vi "Set One Test.vi"() -> ()   [LabVIEW 2018]
doc: "Use this template to build a user interface event handler design pattern. Use this pattern for dialog boxes and other user interfaces. You also can create and execute user-defined events that the VI can handle the same way as user interface events."
uses:
  Private/Types/MALT CardTypes.ctl
panel:
  in  "State":bool
  in  "Port":i32=4
  in  "Address":i32=3
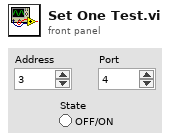
[diagram p1: front panel]
types:
  T1 = typedef "MALT CardTypes.ctl" = enum32{"-", "YAV90832", "YAV904X8", "MALT132", "YAV91616", "YAV90PIN", "YAV90096", "YAV90HVT", "YAV90CLR", "YAV90128", "YAV90PNE", "YAVCANCON", "YAV91775", "YAV90XXX", "YAV90MMU", "H730050", "H710060", "H710061", "YAV90304", "MMI", "YAV90060", "MALT160T", "YAV90059", "Not Defined"}
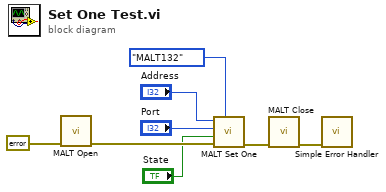
[diagram p0: block diagram]
diagram:
  n1 = call "MALT Open.vi"("error in"=errorcluster {"status"=FALSE, "code"=0, "source"=""}) -> ("error out"=w8:errorcluster)  [unwired: 10 in]
  n2 = call "MALT Set One.vi"("MALT FamilyCode"=MALT_CardTypes."MALT132" ("MALT CardType"), "error in"=w8, "State"="State", "Relay Num"="Port", "Address"="Address") -> ("error out"=w2:errorcluster)  [unwired: 5 in]
  n3 = call "MALT Close.vi"("error in"=w2) -> ("error out"=w6:errorcluster)  [unwired: 10 in]
  n4 = call <vilib>:"Simple Error Handler.vi"("error in (no error)"=w6) -> ()  [unwired: 4 in, 5 out]
